vi "Main.vi"(8 "error in":errorcluster, 11 "Servo Motor Emulator in":refnum<class "Servo Motor Emulator.lvclass">) -> (0 "error out":errorcluster, 3 "Servo Motor Emulator out":refnum<class "Servo Motor Emulator.lvclass">)   [LabVIEW 2017, in "Servo Motor Emulator.lvclass"]
doc: "The <b>Queued Message Handler</b> of the Worker that owns this VI."
uses:
  Servo Motor Emulator.lvclass
  C:/Program Files (x86)/National Instruments/LabVIEW 2017/vi.lib/addons/_Workers/Library/Classes/Worker/Worker.lvclass
  Initialization Data.ctl
  Response Cases.ctl
  <vilib>/addons/_Workers/Library/Case Label.ctl
  Servo Motor Emulator.lvclass/Servo Motor Emulator.ctl
  rql_Humidity Changed.ctl
  rsp_Report Humidity.ctl
  rql_Temperature Changed.ctl
  rsp_Report Temperature.ctl
  rqp_Set Position.ctl
  <vilib>/addons/_Workers/Library/Classes/Message Queue/Message Queue.lvclass
  <vilib>/addons/_Workers/Library/Workers.lvlib
panel:
  in  "RH":dbl
  in  "Temperature":dbl
  out "Position":dbl(knob) scale=0.0..180.0
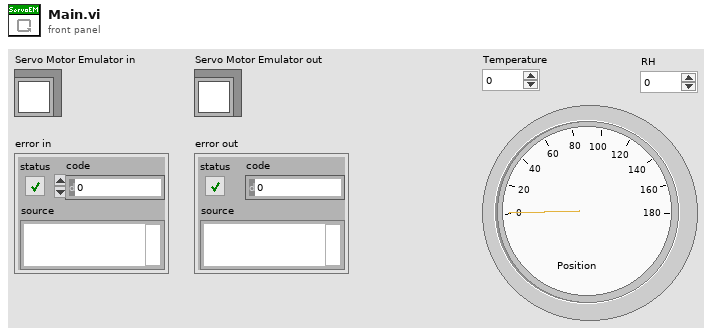
[diagram p1: front panel]
types:
  T1 = typedef "Servo Motor Emulator.lvclass/Initialization Data.ctl" = cluster{"Response Cases":T2}
  T2 = typedef "Servo Motor Emulator.lvclass/Response Cases.ctl" = cluster{"Report Temperature":T3, "Report Humidity":T3}
  T3 = typedef "Workers.lvlib/Case Label.ctl" = string
  T4 = typedef "Servo Motor Emulator.lvclass/rsp_Report Humidity.ctl" = cluster{"Humidity":dbl}
  T5 = typedef "Servo Motor Emulator.lvclass/rql_Humidity Changed.ctl" = cluster{"Placeholder":string}
  T6 = typedef "Servo Motor Emulator.lvclass/rsp_Report Temperature.ctl" = cluster{"Temperature":dbl}
  T7 = typedef "Servo Motor Emulator.lvclass/rql_Temperature Changed.ctl" = cluster{"Placeholder":string}
  T8 = typedef "Servo Motor Emulator.lvclass/rqp_Set Position.ctl" = cluster{"Position":dbl}
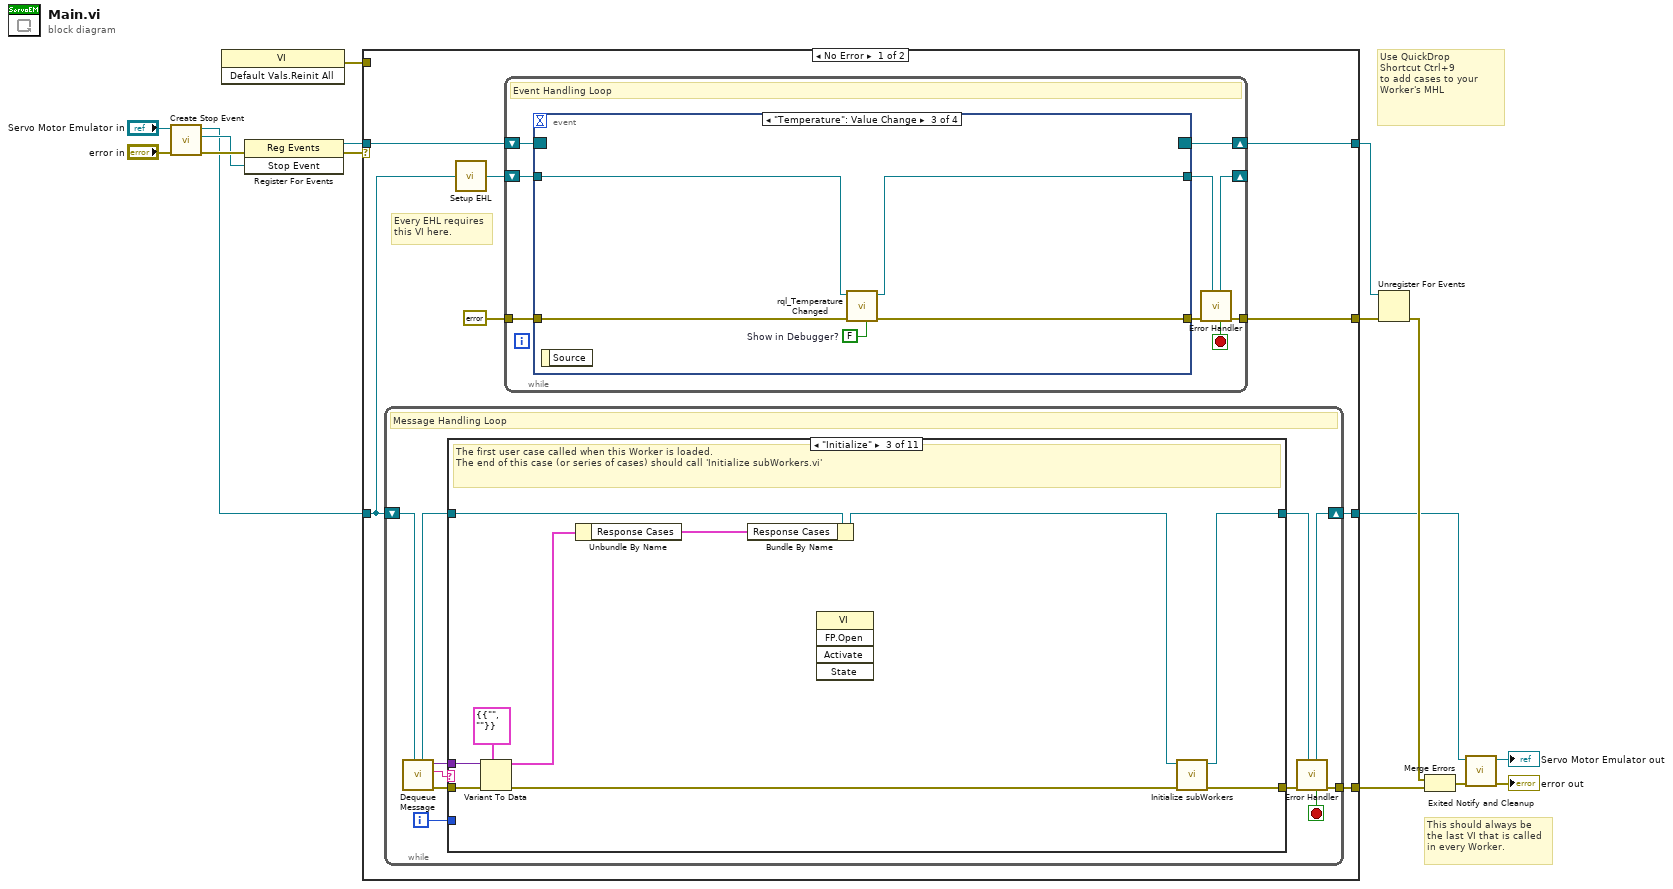
[diagram p0: block diagram]
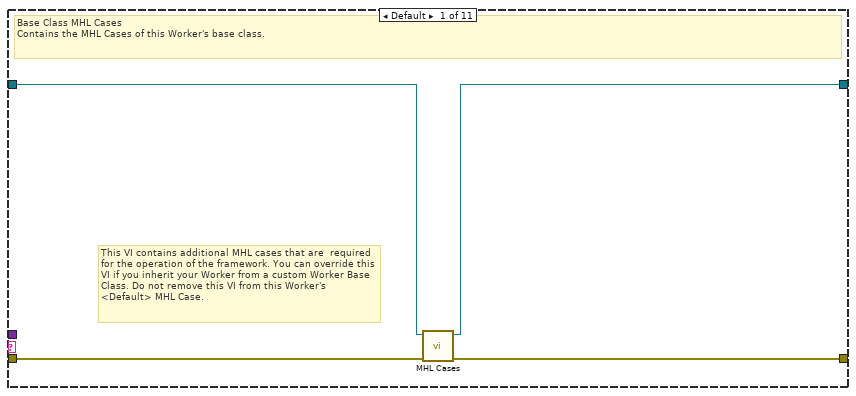
[diagram p2: hidden frame]
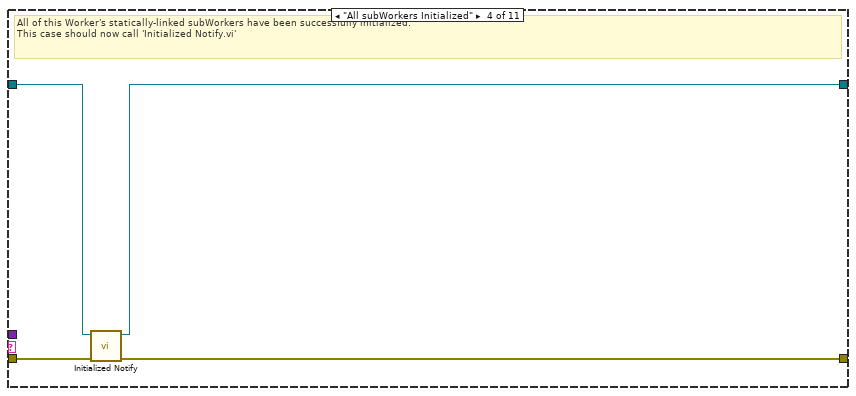
[diagram p4: hidden frame]
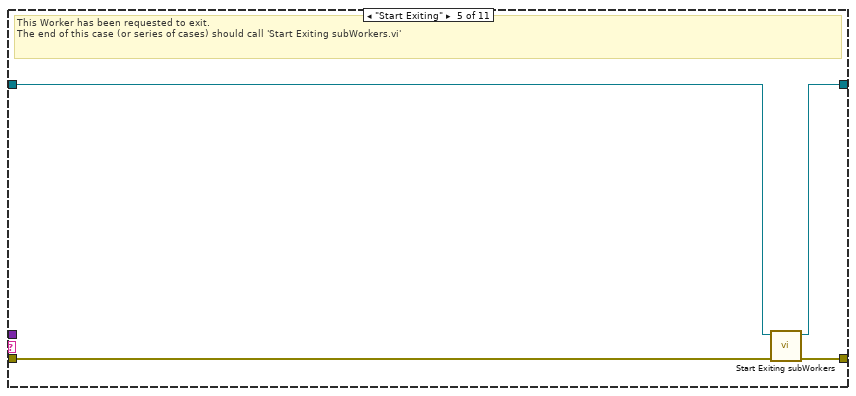
[diagram p5: hidden frame]
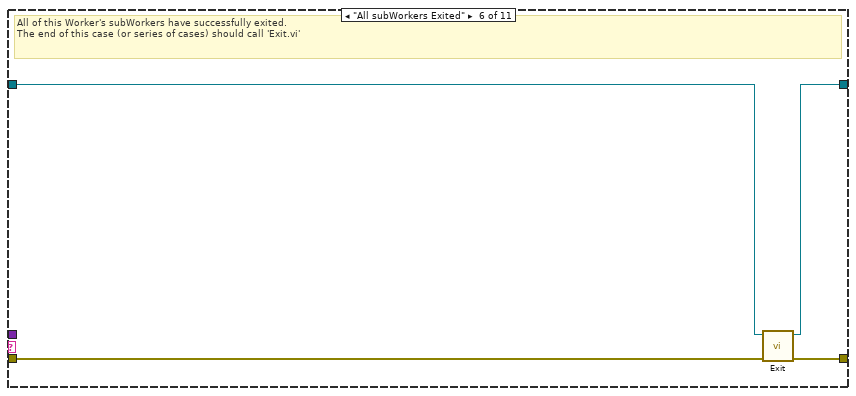
[diagram p6: hidden frame]
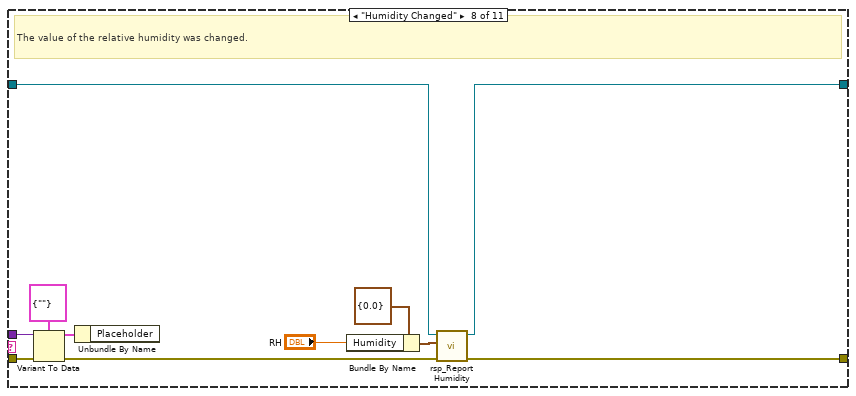
[diagram p8: hidden frame]
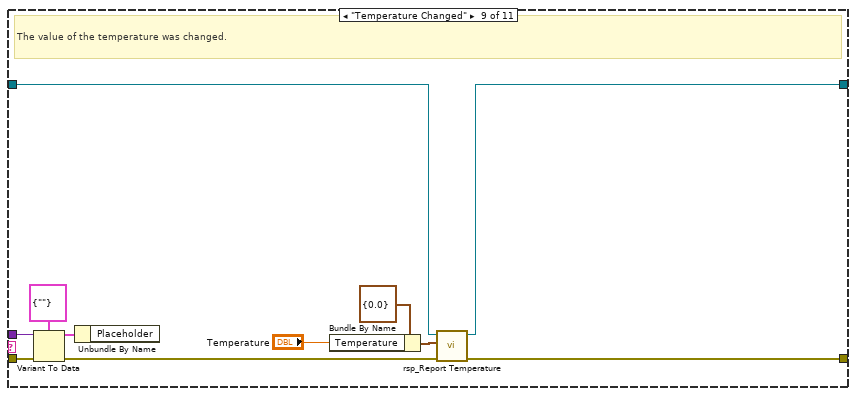
[diagram p9: hidden frame]
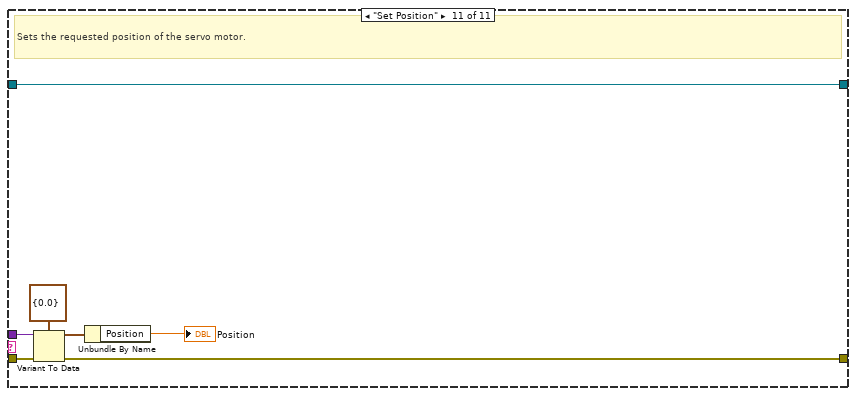
[diagram p11: hidden frame]
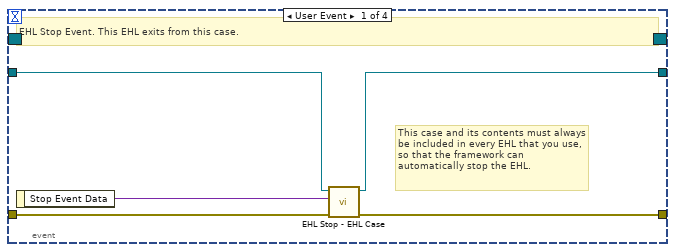
[diagram p12: hidden frame]
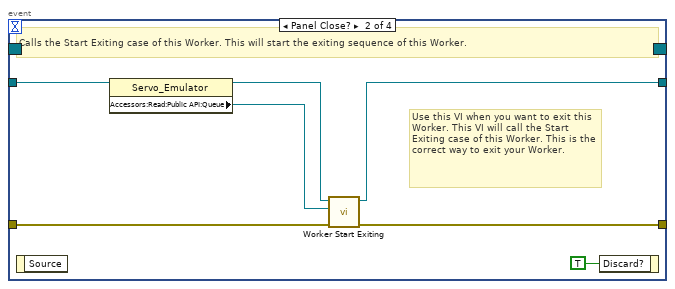
[diagram p13: hidden frame]
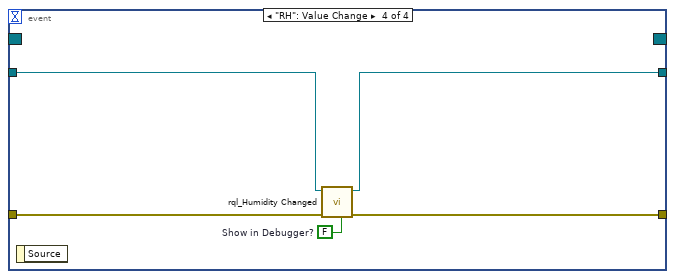
[diagram p14: hidden frame]
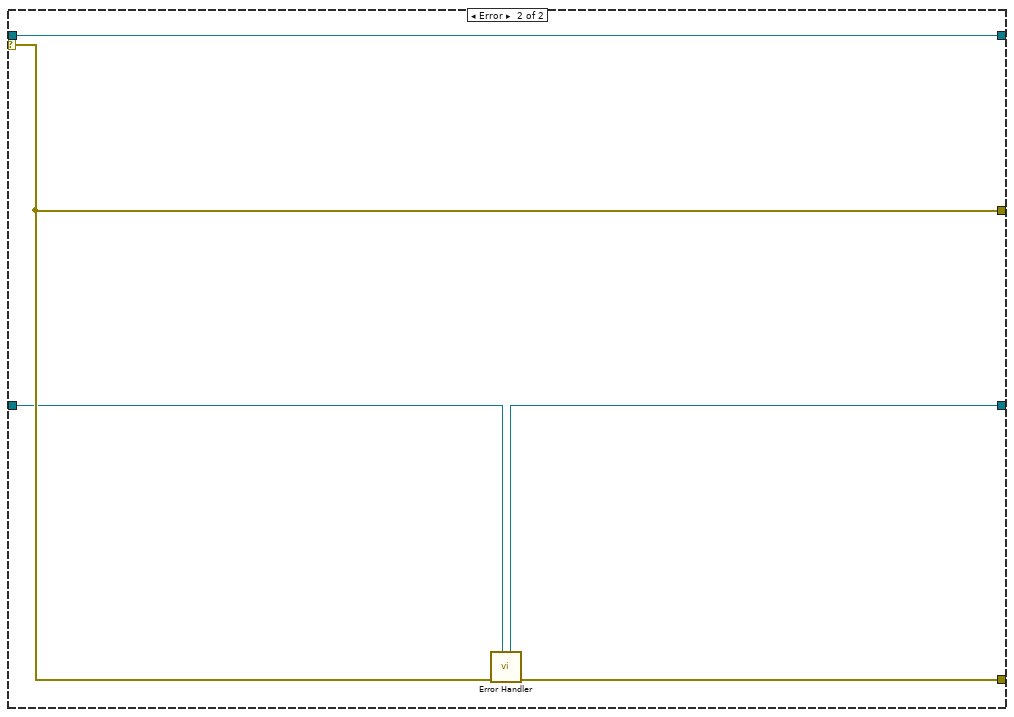
[diagram p15: hidden frame]
diagram:
  # "Use QuickDrop\nShortcut Ctrl+9\nto add cases to your\nWorker's MHL"
  # "This should always be the last VI that is called in every Worker."
  n1 = call-dynamic "Create Stop Event.vi"("error in"="error in", "Worker"="Servo Motor Emulator in") -> ("error out"=w11:errorcluster, "Stop Event"=w8:refnum<user-event>, "Worker out"=w5:refnum<class "Servo Motor Emulator.lvclass">)  [unwired: 7 in]
  n2 = invoke class="VI" method="Default Vals.Reinit All"() -> (error out=w1:errorcluster)  [unwired: 3 in, 2 out]
  n3 = register-events(error in=w11, w8) -> (reference out=w10:refnum<event-registration>, error out=w2:errorcluster)  [unwired: 1 in]
  n4 = case shown="No Error" w2 {
    tunnel: w5 -> [w19 w129]
    tunnel: [w17 w130] -> w9
    tunnel: w10 -> [w24 w131]
    tunnel: [w21 w132] -> w15
    tunnel: [w23 w131] -> w14
    tunnel: [w18 w128] -> w12
    selector: w2 -> [_ w132]
    tunnel: w1 -> [_ _]
    frame No Error {
      # "Every EHL requires\nthis VI here."
      n5 = while {
        shift-right: [w33] -> w18
        shift-left: w19 -> [w35]
        tunnel: [w34] -> w17
        i -> [w26]
        stop <- w27 stop-if-true
        # "Message Handling Loop"
        n6 = call-dynamic "Dequeue Message.vi"("Worker"=w35) -> ("error out"=w32:errorcluster, "Case out"=w28:string, "Data out"=w25:variant, "Worker out"=w30:refnum<class "Servo Motor Emulator.lvclass">)  [unwired: 6 in, 1 out]
        n7 = case "Worker MHL Case Structure (DO NOT CHANGE LABEL NAME)" shown="\"Initialize\"" w28 {
          tunnel: w32 -> [w39 w40 w49 w53 w56 w63 w65 w76 w87 w89 w95]
          tunnel: [w38 w40 w51 w52 w59 w62 w65 w71 w82 w89 w94] -> w31
          tunnel: w30 -> [w37 w41 w48 w55 w57 w61 w64 w70 w81 w88 w96]
          tunnel: [w36 w41 w50 w54 w58 w60 w64 w69 w80 w88 w96] -> w29
          tunnel: w26 -> [_ _ _ _ _ _ _ _ _ _ _]
          tunnel: w25 -> [_ _ w46 _ _ _ _ w73 w84 _ w92]
          frame Default {
            # "This VI contains additional MHL cases that are  required for the operation of the framework. You can override this VI if you inherit your Worker from a custom Worker Base Class. Do not remove this VI from this Worker's <Default> MHL Case."
            # "Base Class MHL Cases\nContains the MHL Cases of this Worker's base class."
            n8 = call-dynamic "MHL Cases.vi"("error in"=w39, "Worker in"=w37) -> ("error out"=w38:errorcluster, "Worker out"=w36:refnum<class "Servo Motor Emulator.lvclass">)  [unwired: 8 in]
          }
          frame "------------ FRAMEWORK CASES -----------" {
            # "Start of Workers Framework Cases"
          }
          frame "Initialize" {
            # "The first user case called when this Worker is loaded.\nThe end of this case (or series of cases) should call 'Initialize subWorkers.vi'"
            n9 = Variant To Data(error in=w49, type=T1 {"Response Cases"={"Report Temperature"="", "Report Humidity"=""}} ("Initialization Data"), Variant=w46) -> (data=w44:T1, error out=w47:errorcluster)
            n10 = Unbundle By Name(w44) -> ("Response Cases"=w43:T2)
            n11 = Bundle By Name(cluster=w48, "Response Cases"=w43) -> (w45:refnum<class "Servo Motor Emulator.lvclass">)
            n12 = invoke class="VI" method="FP.Open"() -> ()  [unwired: 5 in, 5 out]
            n13 = call-dynamic "Initialize subWorkers.vi"("error in"=w47, "Worker"=w45) -> ("error out"=w51:errorcluster, "dup Worker out"=w50:refnum<class "Servo Motor Emulator.lvclass">)  [unwired: 8 in]
          }
          frame "All subWorkers Initialized" {
            # "All of this Worker's statically-linked subWorkers have been successfully initialized.\nThis case should now call 'Initialized Notify.vi'"
            n14 = call-dynamic "Initialized Notify.vi"("error in"=w53, "Worker"=w55) -> ("error out"=w52:errorcluster, "dup Worker out"=w54:refnum<class "Servo Motor Emulator.lvclass">)  [unwired: 8 in]
          }
          frame "Start Exiting" {
            # "This Worker has been requested to exit. \nThe end of this case (or series of cases) should call 'Start Exiting subWorkers.vi'"
            n15 = call-dynamic "Start Exiting subWorkers.vi"("error_in"=w56, "Worker"=w57) -> ("error out"=w59:errorcluster, "dup Worker out"=w58:refnum<class "Servo Motor Emulator.lvclass">)  [unwired: 8 in]
          }
          frame "All subWorkers Exited" {
            # "All of this Worker's subWorkers have successfully exited. \nThe end of this case (or series of cases) should call 'Exit.vi'"
            n16 = call-dynamic "Exit.vi"("error_in"=w63, "Worker"=w61) -> ("error out"=w62:errorcluster, "dup Worker out"=w60:refnum<class "Servo Motor Emulator.lvclass">)  [unwired: 8 in]
          }
          frame "------------- LOCAL API CASES -------------" {
            # "Start of Workers Local API Cases"
          }
          frame "Humidity Changed" {
            # "The value of the relative humidity was changed."
            n17 = Variant To Data(error in=w76, type=T5 {"Placeholder"=""} ("Data"), Variant=w73) -> (data=w72:T5, error out=w75:errorcluster)
            n18 = Unbundle By Name(w72) -> ()  [unwired: 1 out]
            n19 = Bundle By Name(cluster=T4 {"Humidity"=0.0} ("Data in"), "Humidity"="RH") -> (w67:T4)
            n20 = call "rsp_Report Humidity.vi"("error in"=w75, "Data in"=w67, "Servo Motor Emulator in"=w70) -> ("error out"=w71:errorcluster, "dup Servo Motor Emulator out"=w69:refnum<class "Servo Motor Emulator.lvclass">)  [unwired: 7 in]
          }
          frame "Temperature Changed" {
            # "The value of the temperature was changed."
            n21 = Variant To Data(error in=w87, type=T7 {"Placeholder"=""} ("Data"), Variant=w84) -> (data=w83:T7, error out=w86:errorcluster)
            n22 = Unbundle By Name(w83) -> ()  [unwired: 1 out]
            n23 = Bundle By Name(cluster=T6 {"Temperature"=0.0} ("Data in"), "Temperature"="Temperature") -> (w78:T6)
            n24 = call "rsp_Report Temperature.vi"("error in"=w86, "Data in"=w78, "Servo Motor Emulator in"=w81) -> ("error out"=w82:errorcluster, "dup Servo Motor Emulator out"=w80:refnum<class "Servo Motor Emulator.lvclass">)  [unwired: 7 in]
          }
          frame "------------- PUBLIC API CASES -------------" {
            # "Start of Workers Public API Cases"
          }
          frame "Set Position" {
            # "Sets the requested position of the servo motor."
            n25 = Variant To Data(error in=w95, type=T8 {"Position"=0.0} ("Data"), Variant=w92) -> (data=w91:T8, error out=w94:errorcluster)
            n26 = Unbundle By Name(w91) -> ("Position"=→"Position":dbl)
          }
        }
        n27 = call-dynamic "Error Handler.vi"("Worker"=w29, "error_in"=w31) -> ("error out"=w34:errorcluster, "Stop Loop"=w27:bool, "Worker out"=w33:refnum<class "Servo Motor Emulator.lvclass">)  [unwired: 7 in]
      }
      n28 = call-dynamic "Setup EHL.vi"("Worker"=w19) -> ("Worker out"=w20:refnum<class "Servo Motor Emulator.lvclass">)  [unwired: 14 in]
      n29 = while "Event Handling Loop" {
        shift-right: [w105] -> w23
        shift-left: w24 -> [w104]
        tunnel: [w100] -> w21
        tunnel: errorcluster {"status"=FALSE, "code"=0, "source"=""} ("error constant") -> [w102]
        shift-right: [w98] -> _
        shift-left: w20 -> [w103]
        stop <- w97 stop-if-true
        # "Event Handling Loop"
        n30 = event shown="[2] \"Temperature\": Value Change" {
          selector: w104 -> [_ _ _ _]
          dyn-events: [_ _ _ _] -> w105
          timeout: _ -> [_ _ _ _]
          tunnel: [w109 w116 w121 w126] -> w101
          tunnel: w102 -> [w110 w115 w122 w127]
          tunnel: w103 -> [w108 w114 w120 w125]
          tunnel: [w107 w113 w119 w124] -> w99
          event User Event {
            # "This case and its contents must always be included in every EHL that you use, so that the framework can automatically stop the EHL."
            # "EHL Stop Event. This EHL exits from this case."
            n31 = event-data() -> ("Stop Event Data"=w106:variant)  [unwired: 1 in]
            n32 = call-dynamic "EHL Stop - EHL Case.vi"("error in"=w110, "Stop Event Data"=w106, "Worker"=w108) -> ("error out"=w109:errorcluster, "Worker out"=w107:refnum<class "Servo Motor Emulator.lvclass">)  [unwired: 7 in]
          }
          event Panel Close? {
            # "Use this VI when you want to exit this Worker. This VI will call the Start Exiting case of this Worker. This is the correct way to exit your Worker."
            # "Calls the Start Exiting case of this Worker. This will start the exiting sequence of this Worker."
            n33 = event-data() -> ()  [unwired: 1 in, 1 out]
            n34 = property class="Servo_Emulator"(reference=w114) -> (reference out=w112:refnum<class "Servo Motor Emulator.lvclass">, "Accessors:Read:Public API:Queue"=w111:refnum<class "Message Queue.lvclass">)  [unwired: 1 in, 1 out]
            n35 = call-dynamic "Worker Start Exiting.vi"("error_in"=w115, "Message Queue"=w111, "Worker"=w112) -> ("error out"=w116:errorcluster, "dup Worker out"=w113:refnum<class "Servo Motor Emulator.lvclass">)  [unwired: 7 in]
            n36 = event-data("Discard?"=TRUE) -> ()  [unwired: 1 in, 1 out]
          }
          event "Temperature": Value Change {
            w118 = FALSE  # Show in Debugger?
            n37 = event-data() -> ()  [unwired: 1 in, 1 out]
            n38 = call "rql_Temperature Changed.vi"("Show in Debugger?"=w118, "error in"=w122, "Servo Motor Emulator in"=w120) -> ("error out"=w121:errorcluster, "dup Servo Motor Emulator out"=w119:refnum<class "Servo Motor Emulator.lvclass">)  [unwired: 7 in]
          }
          event "RH": Value Change {
            w123 = FALSE  # Show in Debugger?
            n39 = event-data() -> ()  [unwired: 1 in, 1 out]
            n40 = call "rql_Humidity Changed.vi"("Show in Debugger?"=w123, "error in"=w127, "Servo Motor Emulator in"=w125) -> ("error out"=w126:errorcluster, "dup Servo Motor Emulator out"=w124:refnum<class "Servo Motor Emulator.lvclass">)  [unwired: 7 in]
          }
        }
        n41 = call-dynamic "Error Handler.vi"("Worker"=w99, "error_in"=w101) -> ("error out"=w100:errorcluster, "Stop Loop"=w97:bool, "Worker out"=w98:refnum<class "Servo Motor Emulator.lvclass">)  [unwired: 7 in]
      }
    }
    frame Error {
      n42 = call-dynamic "Error Handler.vi"("Worker"=w129, "error_in"=w132) -> ("error out"=w130:errorcluster, "Worker out"=w128:refnum<class "Servo Motor Emulator.lvclass">)  [unwired: 7 in, 1 out]
    }
  }
  n43 = Unregister For Events(event registration refnum=w14, error in=w15) -> (error out=w16:errorcluster)
  n44 = Merge Errors(w16, w9) -> (w13:errorcluster)
  n45 = call-dynamic "Exited Notify and Cleanup.vi"("error_in"=w13, "Worker"=w12) -> ("error out"=→"error out":errorcluster, "dup Worker out"=→"Servo Motor Emulator out":refnum<class "Servo Motor Emulator.lvclass">)  [unwired: 8 in]
